vi "Close_Connection.vi"(8 "error in (no error)":errorcluster, 11 "Simulated uC in":refnum<class "Simulated uC.lvclass">) -> (0 "error out":errorcluster, 3 "Simulated uC out":refnum<class "Simulated uC.lvclass">)   [LabVIEW 2019, in "Simulated uC.lvclass"]
uses:
  Simulated uC.lvclass
  Clase Padre/Serial Device.lvclass
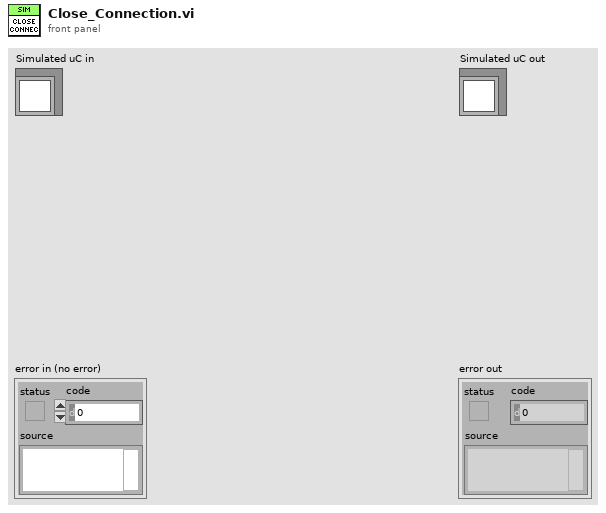
[diagram p1: front panel]
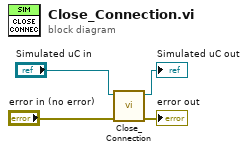
[diagram p0: block diagram]
diagram:
  n1 = call-parent "Close_Connection.vi"("error in (no error)"="error in (no error)", "Serial Device in"="Simulated uC in") -> ("error out"=→"error out":errorcluster, "Serial Device out"=→"Simulated uC out":refnum<class "Simulated uC.lvclass">)  [unwired: 8 in]
